vi "Update Static Overlay.vi"(8 "error in (no error)":errorcluster, 10 "Static Overlay":refnum<class "Static Overlay.lvclass">, 11 "HIJ Vision Display in":refnum<class "HIJ Vision Display.lvclass">) -> (0 "error out":errorcluster, 3 "HIJ Vision Display out":refnum<class "HIJ Vision Display.lvclass">)   [LabVIEW 2014, in "HIJ Vision Display.lvlib" / "HIJ Vision Display.lvclass"]
uses:
  HIJ Vision Display.lvclass
  Analyze/Results and Overlays/Static Overlay/Static Overlay.lvclass
  HIJ Vision Display.lvclass/HIJ Vision Display.ctl
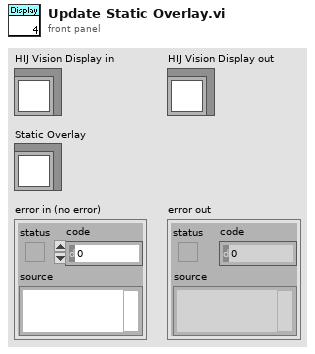
[diagram p1: front panel]
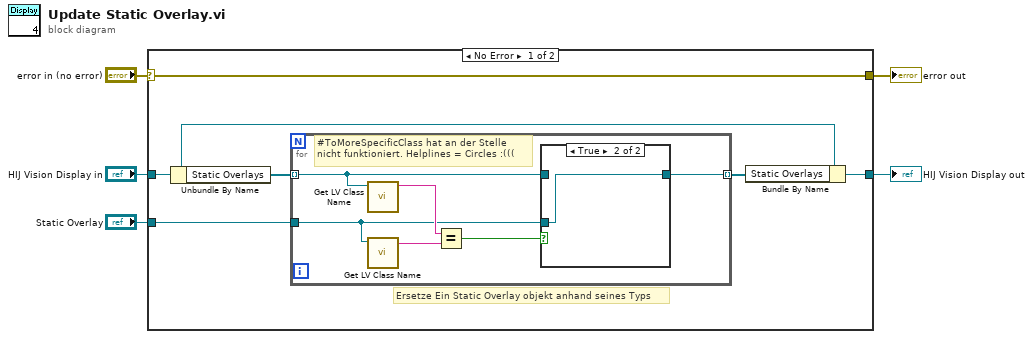
[diagram p0: block diagram]
diagram:
  n1 = case shown="No Error" "error in (no error)" {
    selector: "error in (no error)" -> [w11 w21]
    tunnel: [w11 w21] -> w4
    tunnel: [w9 w20] -> w2
    tunnel: "HIJ Vision Display in" -> [w10 w20]
    tunnel: "Static Overlay" -> [w8 _]
    frame No Error {
      # "Ersetze Ein Static Overlay objekt anhand seines Typs"
      n2 = Unbundle By Name(w10) -> ("Static Overlays"=w7:refnum<class "Static Overlay.lvclass">[])
      n3 = for {
        tunnel: w8 -> [w12]
        tunnel: w7 -> [w16] mode=indexing
        tunnel: [w17] -> w6 mode=indexing
        # "#ToMoreSpecificClass hat an der Stelle\nnicht funktioniert. Helplines = Circles :((("
        n4 = call <vilib>:"Get LV Class Name.vi"("object"=w16) -> ("class name"=w15:string)  [unwired: 9 in, 1 out]
        n5 = call <vilib>:"Get LV Class Name.vi"("object"=w12) -> ("class name"=w14:string)  [unwired: 9 in, 1 out]
        n6 = Equal?(x=w15, y=w14) -> (x = y?=w13:bool)
        n7 = case shown="True" w13 {
          tunnel: [w18 w19] -> w17
          tunnel: w16 -> [w18 _]
          tunnel: w12 -> [_ w19]
          frame False {
          }
          frame True {
          }
        }
      }
      n8 = Bundle By Name(cluster=w10, "Static Overlays"=w6) -> (w9:refnum<class "HIJ Vision Display.lvclass">)
    }
    frame Error {
    }
  }
  "error out" <- w4
  "HIJ Vision Display out" <- w2
